vi "GlobalRhPercent.vi"() -> ()   [LabVIEW 2014]
panel:
  out "Rh Global":dbl
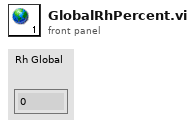
[diagram p1: front panel]
diagram:
